vi "nm_eV.vi"(7 "nm":dbl) -> (8 "eV":dbl)   [LabVIEW 2023]
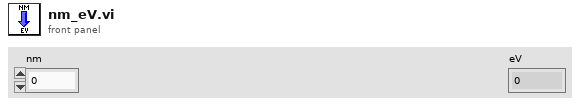
[diagram p1: front panel]
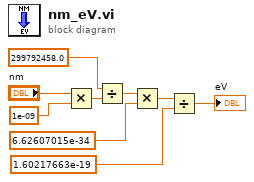
[diagram p0: block diagram]
diagram:
  n1 = Multiply(x="nm", y=1e-09) -> (x*y=w7:dbl)
  n2 = Divide(x=299792458.0, y=w7) -> (x/y=w5:dbl)
  n3 = Multiply(x=w5, y=6.62607015e-34) -> (x*y=w3:dbl)
  n4 = Divide(x=w3, y=1.60217663e-19) -> (x/y=→"eV":dbl)
